vi "Day 6 (Part One).vi"() -> ()   [LabVIEW 2021]
panel:
  out "Position":i32
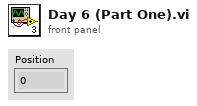
[diagram p1: front panel]
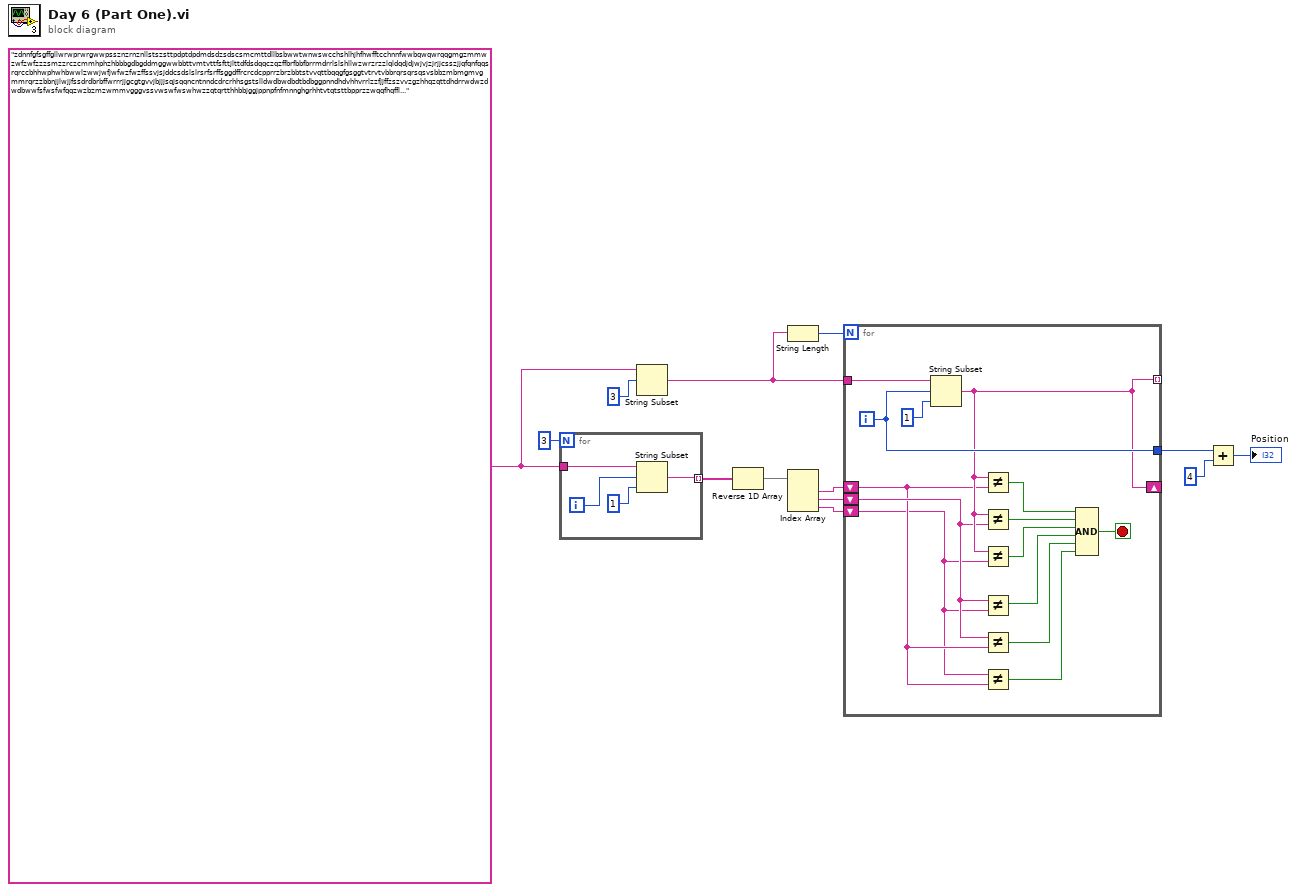
[diagram p0: block diagram]
diagram:
  w13 = "zdnnfgfsgffgllwrwprwrgwwpssznzrnznllstszsttpdptdpdmdsdzsdscsmcmttdllbsbwwtwnwswcchshlhjhfhwfftcchnnfwwbqwqwrqqgmgzmmwzwfzwfzzzsmzzrczcmmhphzhbbbgdbgddmggwwbbttvmtvttfsfttjlttdfdsdqqczqzffbrfbbfbrrmdrrlslshllwzwrzrzzlqldqdjdjwjvjzjrjjcsszjjqfqnfqqsrqrccbhhwphwhbwwlzwwjwfjwfwzfwzffssvjsjddcsdslslrsrfsrffsggdffrcrcdcpprrzbrzbbtstvvqttbqqgfgsggtvtrvtvbbrqrsqrsqsvsbbzmbmgmvgmmrqrzzbbnjjlwjjfssdrdbrbffwrrrjjgcgtgvvjbjjjsqjsqqncntnndcdrcrhhsgstslldwdbwdbdtbdbggpnndhdvhhvrrlzzfjjffzszvvzgzhhqzqttdhdrrwdwzdwdbwwfsfwsfwfqqzwzbzmzwmmvgggvssvwswfwswhwzzqtqrtthhbbjggjppnpfnfmnnghgrhhtvtqtsttbpprzzwqqfhqffl..."
  n1 = for {
    N: 3 -> [_]
    tunnel: w13 -> [w17]
    tunnel: [w14] -> w12 mode=indexing
    i -> [w16]
    n2 = String Subset(string=w17, offset (0)=w16, length (rest)=1 ("length (rest)")) -> (substring=w14:string)
  }
  n3 = String Subset(string=w13, offset (0)=3) -> (substring=w6:string)  [unwired: 1 in]
  n4 = Reverse 1D Array(array=w12) -> (reversed array=w1:string[])
  n5 = String Length(string=w6) -> (length=w5:i32)
  n6 = Index Array(array=w1) -> (element #1=w9:string, element #2=w10:string, element #3=w11:string)  [unwired: 3 in]
  n7 = for {
    N: w5 -> [_]
    shift-right: [w24] -> _
    shift-left: w9 -> [w22]
    shift-left: w10 -> [w23]
    shift-left: w11 -> [w21]
    tunnel: w6 -> [w31]
    tunnel: [w25] -> w4
    tunnel: [w24] -> _ mode=indexing
    i -> [w25]
    stop <- w26 stop-if-true
    n8 = String Subset(string=w31, offset (0)=w25, length (rest)=1 ("length (rest)")) -> (substring=w24:string)
    n9 = Not Equal?(x=w24, y=w22) -> (x != y?=w29:bool)
    n10 = Not Equal?(x=w24, y=w23) -> (x != y?=w28:bool)
    n11 = Not Equal?(x=w24, y=w21) -> (x != y?=w27:bool)
    n12 = Not Equal?(x=w23, y=w21) -> (x != y?=w18:bool)
    n13 = Not Equal?(x=w23, y=w22) -> (x != y?=w19:bool)
    n14 = Not Equal?(x=w21, y=w22) -> (x != y?=w20:bool)
    n15 = Compound Arithmetic op=AND(w29, w28, w27, w18, w19, w20) -> (w26:bool)
  }
  n16 = Add(x=w4, y=4) -> (x+y=→"Position":i32)
